vi "__SW_8710XB_6501.vi"(0 "Path(1..6)":i32=1, 1 "ch(1..6)":i32=4, 2 "bit(4or6)":i32=4, 3 "Dev(1,2..)":i32=1) -> ()   [LabVIEW 2017]
panel:
  out "設定値":i32=15
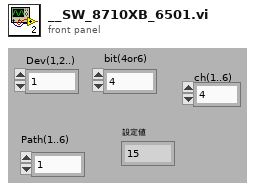
[diagram p1: front panel]
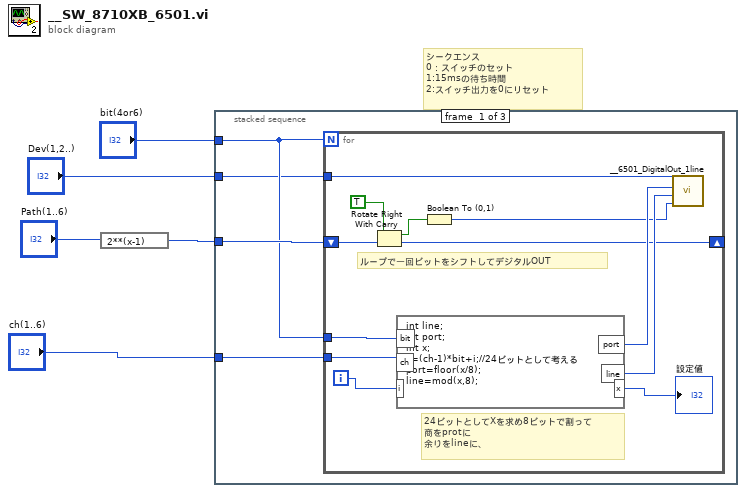
[diagram p0: block diagram]
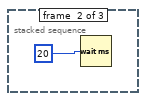
[diagram p2: hidden frame]
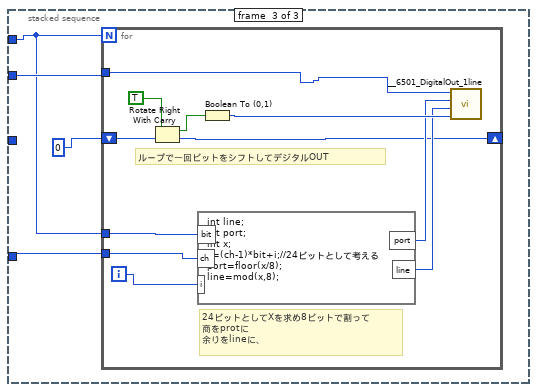
[diagram p3: hidden frame]
diagram:
  # "シークエンス\n0：スイッチのセット\n1:15msの待ち時間\n2:スイッチ出力を0にリセット"
  n1 = expression code="2**(x-1)"("Path(1..6)") -> (w5:i32)
  n2 = stacked-sequence {
    tunnel: w5 -> [w9 _ _]
    tunnel: "bit(4or6)" -> [w8 _ w24]
    tunnel: "ch(1..6)" -> [w7 _ w23]
    tunnel: "Dev(1,2..)" -> [w6 _ w26]
    frame #0 {
      n3 = for {
        N: w8 -> [_]
        shift-right: [w15] -> _
        shift-left: w9 -> [w21]
        tunnel: w8 -> [w14]
        tunnel: w7 -> [w13]
        tunnel: w6 -> [w12]
        i -> [w19]
        # "ループで一回ビットをシフトしてデジタルOUT"
        # "24ビットとしてXを求め8ビットで割って\n商をprotに\n余りをlineに、"
        n4 = Rotate Right With Carry(2:w21, 3:TRUE) -> (0:w15:i32, 1:w20:bool)
        n5 = formula code="int line;\nint port;\nint x;\nx=(ch-1)*bit+i;//24ビットとして考える\nport=floor(x/8);\nline=mod(x,8);"("bit"=w14, "i"=w19, "ch"=w13) -> ("line"=w17:i32, "port"=w16:i32, "x"=→"設定値":i32)
        n6 = Boolean To (0,1)(Boolean=w20) -> (0, 1=w10:i16)
        n7 = call "__6501_DigitalOut_1line.vi"("OFF,ON(0,1)"=w10, "line(0...7)"=w17, "Port(0,1,2)"=w16, "Dev(1,2..)"=w12) -> ()
      }
    }
    frame #1 {
      n8 = Wait (ms)(milliseconds to wait=20) -> ()  [unwired: 1 out]
    }
    frame #2 {
      n9 = for {
        N: w24 -> [_]
        shift-right: [w30] -> _
        shift-left: 0 -> [w37]
        tunnel: w24 -> [w29]
        tunnel: w23 -> [w28]
        tunnel: w26 -> [w27]
        i -> [w34]
        # "ループで一回ビットをシフトしてデジタルOUT"
        # "24ビットとしてXを求め8ビットで割って\n商をprotに\n余りをlineに、"
        n10 = Rotate Right With Carry(2:w37, 3:TRUE) -> (0:w30:i32, 1:w36:bool)
        n11 = formula code="int line;\nint port;\nint x;\nx=(ch-1)*bit+i;//24ビットとして考える\nport=floor(x/8);\nline=mod(x,8);"("bit"=w29, "i"=w34, "ch"=w28) -> ("line"=w32:i32, "port"=w31:i32)
        n12 = Boolean To (0,1)(Boolean=w36) -> (0, 1=w35:i16)
        n13 = call "__6501_DigitalOut_1line.vi"("OFF,ON(0,1)"=w35, "line(0...7)"=w32, "Port(0,1,2)"=w31, "Dev(1,2..)"=w27) -> ()
      }
    }
  }
